vi "MAX31855USB_delay.vi"(8 "error in (no error)":errorcluster, 11 "VISA Refnum in":refnum<visa-resource-name>) -> (0 "error out":errorcluster, 3 "VISA Refnum out":refnum<visa-resource-name>)   [LabVIEW 2014]
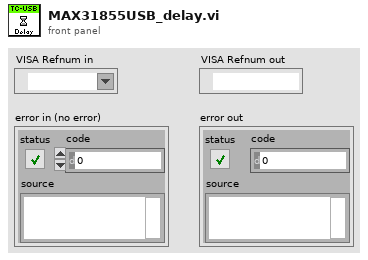
[diagram p1: front panel]
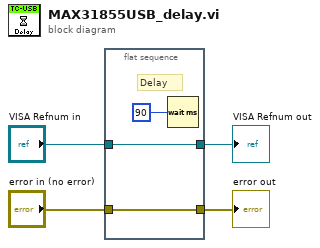
[diagram p0: block diagram]
diagram:
  n1 = flat-sequence {
    tunnel: [w7] -> w4
    tunnel: "VISA Refnum in" -> [w7]
    tunnel: [w6] -> w3
    tunnel: "error in (no error)" -> [w6]
    frame #0 {
      # "Delay"
      n2 = Wait (ms)(milliseconds to wait=u32 90) -> ()  [unwired: 1 out]
    }
  }
  "VISA Refnum out" <- w4
  "error out" <- w3
